vi "End.vi"(8 "error in (no error)":errorcluster, 11 "Acquisition in":refnum<class "Acquisition.lvclass">) -> (0 "error out":errorcluster, 3 "Acquisition out":refnum<class "Acquisition.lvclass">)   [LabVIEW 2018, in "Acquisition.lvclass"]
uses:
  Acquisition.lvclass
  Acquisition.lvclass/Acquisition.ctl
  Comm/Stream/Stream.lvclass
  Channel/Channel.lvclass
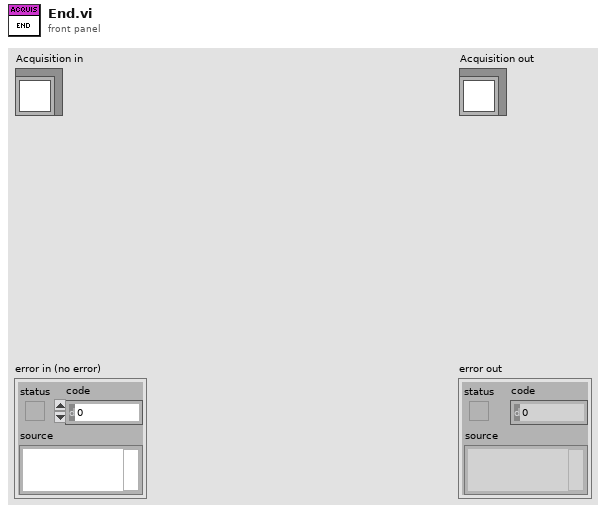
[diagram p1: front panel]
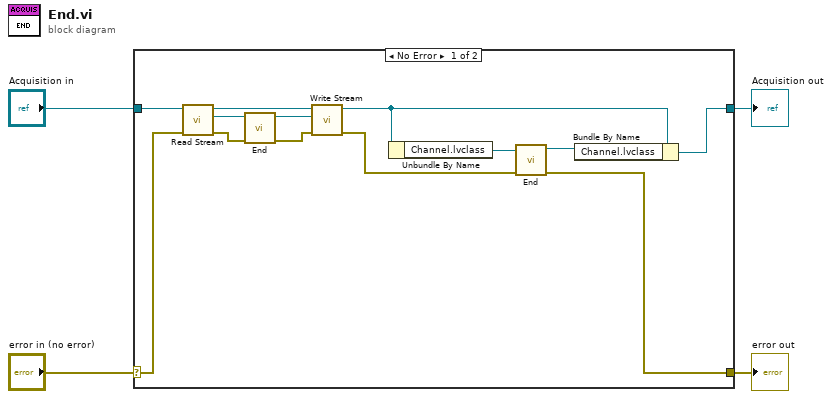
[diagram p0: block diagram]
diagram:
  n1 = case shown="No Error" "error in (no error)" {
    selector: "error in (no error)" -> [w15 w19]
    tunnel: [w5 w19] -> w3
    tunnel: [w7 w18] -> w1
    tunnel: "Acquisition in" -> [w17 w18]
    frame No Error {
      n2 = call-dynamic "Read Stream.vi"("error in (no error)"=w15, "Server in"=w17) -> ("error out"=w14:errorcluster, "Stream.lvclass"=w16:refnum<class "Stream.lvclass">, "Server out"=w11:refnum<class "Acquisition.lvclass">)  [unwired: 7 in]
      n3 = call-dynamic "End.vi"("error in (no error)"=w14, "Stream in"=w16) -> ("error out"=w12:errorcluster, "Stream out"=w13:refnum<class "Stream.lvclass">)  [unwired: 8 in]
      n4 = call-dynamic "Write Stream.vi"("error in (no error)"=w12, "Stream.lvclass"=w13, "Server in"=w11) -> ("error out"=w6:errorcluster, "Server out"=w9:refnum<class "Acquisition.lvclass">)  [unwired: 7 in]
      n5 = Unbundle By Name(w9) -> ("Channel.lvclass"=w10:refnum<class "Channel.lvclass">)
      n6 = call-dynamic "End.vi"("error in (no error)"=w6, "Channel in"=w10) -> ("error out"=w5:errorcluster, "Channel out"=w8:refnum<class "Channel.lvclass">)  [unwired: 8 in]
      n7 = Bundle By Name(cluster=w9, "Channel.lvclass"=w8) -> (w7:refnum<class "Acquisition.lvclass">)
    }
    frame Error {
    }
  }
  "error out" <- w3
  "Acquisition out" <- w1
